vi "NiFPGA Open.vi"(7 "Attribute":T1, 8 "error in (no error)":errorcluster, 9 "Resource":string, 10 "Signature":string, 11 "Bitfile":string) -> (0 "error out":errorcluster, 3 "Session Out":u32)   [LabVIEW 2010, in "FPGA Interface Wrapper.lvlib"]
doc: "Opens a session to the FPGA. This call ensures that the contents of the bitfile are programmed to the FPGA. The FPGA runs unless the NiFpga_OpenAttribute_NoRun attribute is used. Because different operating systems have different default current working directories for applications, you must pass an absolute path for the bitfile parameter. If you pass only the filename instead of an absolute path, the operating system may not be able to locate the bitfile. For example, the default current working directories are C:\\ni-rt\\system\\ for Phar Lap ETS and /c/ for VxWorks. Because the generated *_Bitfile constant is a #define to a string literal, you can use C/C++ string-literal concatenation to form an absolute path. For example, if the bitfile is in the root directory of a Phar Lap ETS system, pass the following for the bitfile parameter. \"C:\\\\\" NiFpga_MyApplication_Bitfile"
uses:
  <userlib>/_FPGA Interface Advanced Tools/FPGA Interface Wrapper/FPGA Interface Wrapper.lvlib
  <userlib>/_FPGA Interface Advanced Tools/FPGA Interface Wrapper/TypeDefs/Open Attribute.ctl
  NiFpga.dll
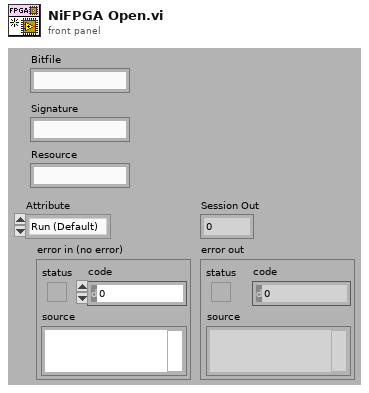
[diagram p1: front panel]
types:
  T1 = typedef "FPGA Interface Wrapper.lvlib/Open Attribute.ctl" = enum32{"Run (Default)", "No Run"}
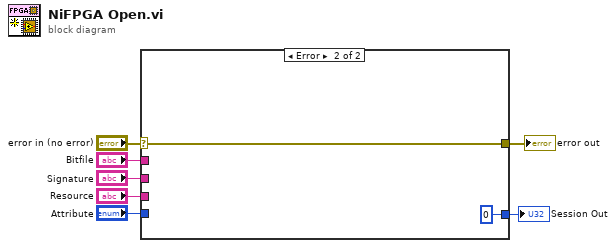
[diagram p0: block diagram]
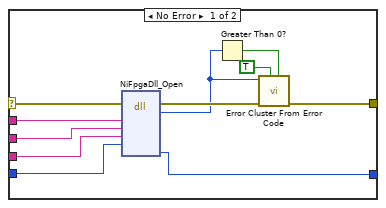
[diagram p2: hidden frame]
diagram:
  n1 = case shown="Error" "error in (no error)" {
    selector: "error in (no error)" -> [w18 w20]
    tunnel: [w9 w20] -> w6
    tunnel: [w17 u32 0 ("Session")] -> w5
    tunnel: "Attribute" -> [w16 _]
    tunnel: "Resource" -> [w15 _]
    tunnel: "Signature" -> [w14 _]
    tunnel: "Bitfile" -> [w13 _]
    frame No Error {
      n2 = dll-call lib="NiFpga.dll" fn="NiFpgaDll_Open"(error in=w18, "Bitfile"=w13, "Signature"=w14, "Resource"=w15, "Attribute"=w16) -> (error out=w10:errorcluster, "Status"=w8:i32, "Session"=w17:u32)  [unwired: 7 in, 1 out]
      n3 = Greater Than 0?(x=w8) -> (x > 0?=w11:bool)
      n4 = call <vilib>:"Error Cluster From Error Code.vi"("is warning? (False)"=w11, "show call chain? (False)"=TRUE, "error in (no error)"=w10, "error code (0)"=w8) -> ("error out"=w9:errorcluster)  [unwired: 5 in]
    }
    frame Error {
    }
  }
  "error out" <- w6
  "Session Out" <- w5
